vi "cluster.vi"() -> ()   [LabVIEW 2017]
panel:
  in  "Cluster 2":cluster{}
  in  "Boolean":bool
  in  "Cluster":T1
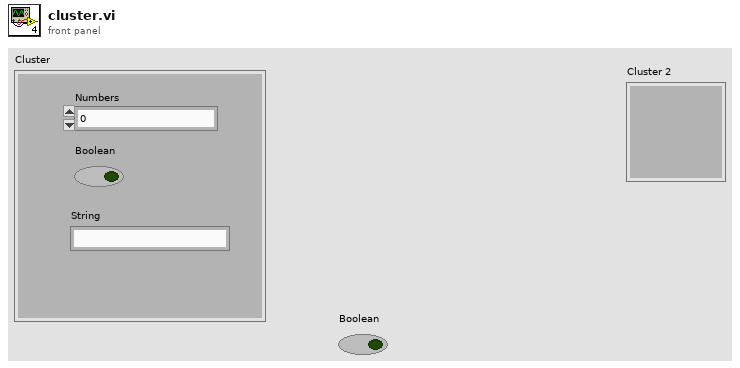
[diagram p1: front panel]
types:
  T1 = cluster{"Numbers":dbl, "Boolean":bool, "String":string}
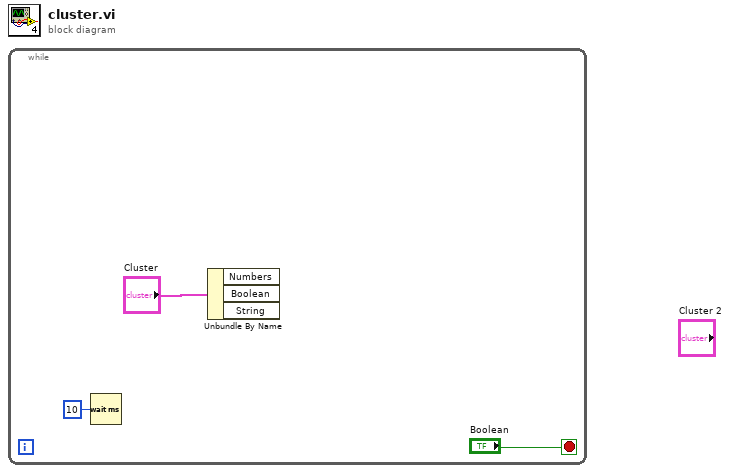
[diagram p0: block diagram]
diagram:
  n1 = while {
    stop <- "Boolean" stop-if-true
    n2 = Wait (ms)(milliseconds to wait=u32 10) -> ()  [unwired: 1 out]
    n3 = Unbundle By Name("Cluster") -> ()  [unwired: 3 out]
  }
